vi "Write Fix.vi"(8 "error in (no error)":errorcluster, 10 "Fix":T1, 11 "DB in":refnum<class "DB.lvclass">) -> (0 "error out":errorcluster, 3 "DB out":refnum<class "DB.lvclass">)   [LabVIEW 2018, in "DB.lvclass"]
uses:
  DB.lvclass
  Def_fix_sql_param.ctl
  DB.lvclass/DB.ctl
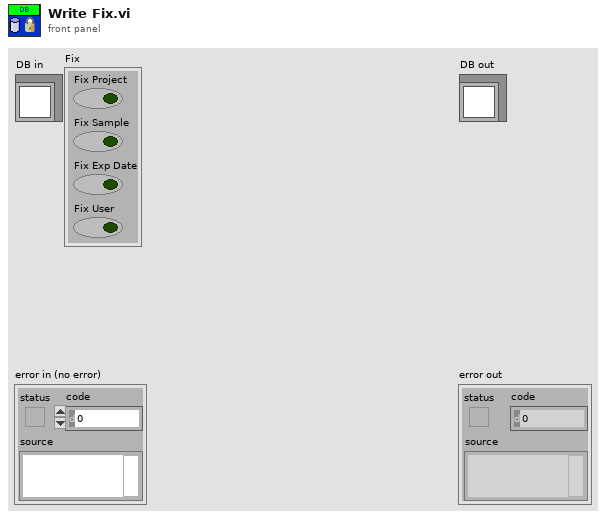
[diagram p1: front panel]
types:
  T1 = typedef "DB.lvclass/Def_fix_sql_param.ctl" = cluster{"Fix Project":bool, "Fix Sample":bool, "Fix Exp Date":bool, "Fix User":bool}
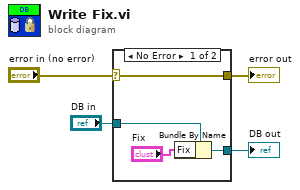
[diagram p0: block diagram]
diagram:
  n1 = case shown="No Error" "error in (no error)" {
    selector: "error in (no error)" -> [w8 w9]
    tunnel: [w8 w9] -> w3
    tunnel: [w6 w10] -> w1
    tunnel: "DB in" -> [w7 w10]
    frame No Error {
      n2 = Bundle By Name(cluster=w7, "Fix"="Fix") -> (w6:refnum<class "DB.lvclass">)
    }
    frame Error {
    }
  }
  "error out" <- w3
  "DB out" <- w1
